vi "Tree.Update.vi"(8 "error in (no error)":errorcluster, 9 "Analysis Tags":string[](array[string]), 10 "Result":bool[](array[boolean]), 11 "TreeControl in":refnum<vi>) -> (0 "error out":errorcluster, 3 "TreeControl out":refnum<vi>)   [LabVIEW 2014, in "NIAnalysis.lvlib"]
uses:
  NIAnalysis.lvlib
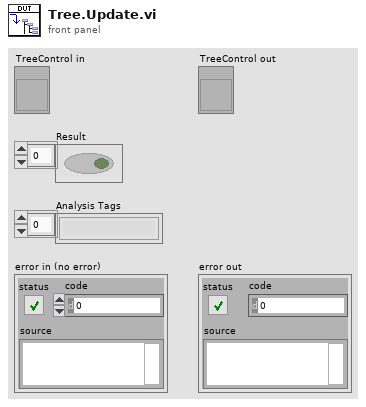
[diagram p1: front panel]
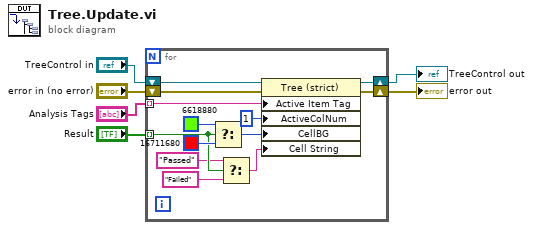
[diagram p0: block diagram]
diagram:
  n1 = for {
    shift-right: [w17] -> w6
    shift-left: "TreeControl in" -> [w18]
    shift-right: [w15] -> w5
    shift-left: "error in (no error)" -> [w16]
    tunnel: "Result" -> [w9] mode=indexing
    tunnel: "Analysis Tags" -> [w14] mode=indexing
    n2 = Select(t=u32 6618880, s=w9, f=u32 16711680) -> (s? t:f=w11:u32)
    n3 = Select(t="Passed", s=w9, f="Failed") -> (s? t:f=w10:string)
    n4 = property class="Tree (strict)"(reference=w18, error in=w16, "Active Item Tag"=w14, "ActiveColNum"=1 ("Active Cell:Active Column Number"), "CellBG"=w11, "Cell String"=w10) -> (reference out=w17:refnum<vi>, error out=w15:errorcluster)
  }
  "TreeControl out" <- w6
  "error out" <- w5
